vi "DoSampleCalibration.vi"(8 "Error In":errorcluster, 10 "TLCamera reference in":refnum<k24>, 11 "MotorController in":refnum<class "MotorController.lvclass">) -> (0 "Error Out":errorcluster, 2 "TLCamera reference out":refnum<k24>, 3 "MotorController out":refnum<class "MotorController.lvclass">)   [LabVIEW 2019]
uses:
  MotorController.lvclass
  C:/Users/jleeman/git_repos/CAxis_Machine/C-Axis LabView Controller/Library_X64/Thorlabs.TSI.TLCameraInterfaces.dll
  Library_X64/Thorlabs.TSI.TLCameraInterfaces.dll
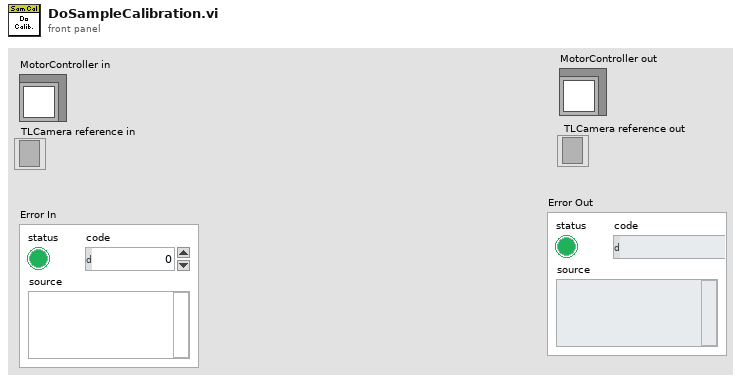
[diagram p1: front panel]
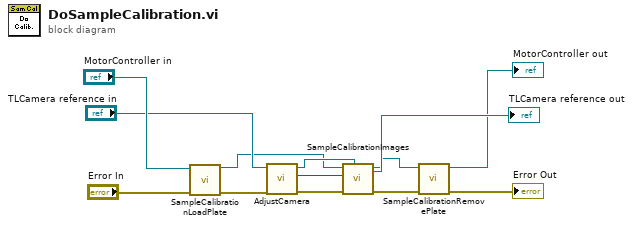
[diagram p0: block diagram]
diagram:
  n1 = call "SampleCalibrationLoadPlate.vi"("Error In"="Error In", "MotorController in"="MotorController in") -> ("Error Out"=w9:errorcluster, "MotorController out"=w5:refnum<class "MotorController.lvclass">)  [unwired: 8 in]
  n2 = call "AdjustCamera.vi"("Error In"=w9, "TLCamera reference in"="TLCamera reference in") -> ("Error Out"=w8:errorcluster, "Exposure (us)"=w4:u32, "TLCamera reference out"=w11:refnum<k24>)  [unwired: 7 in]
  n3 = call "SampleCalibrationImages.vi"("TLCamera reference in"=w11, "Error In"=w8, "ExposureTime_us"=w4, "MotorController in"=w5) -> ("Error Out"=w7:errorcluster, "MotorController out"=w6:refnum<class "MotorController.lvclass">, "TLCamera reference out"=→"TLCamera reference out":refnum<k24>)  [unwired: 5 in]
  n4 = call "SampleCalibrationRemovePlate.vi"("Error In"=w7, "MotorController in"=w6) -> ("Error Out"=→"Error Out":errorcluster, "MotorController out"=→"MotorController out":refnum<class "MotorController.lvclass">)  [unwired: 8 in]
